vi "ReCheckStrips.vi"(0 "Probe Card Channels":i32=32, 5 "Auto Re-Check":bool, 7 "Thresholds":T1, 9 "Bad channel list":i32[](array[numeric]), 10 "region in":u32, 11 "Number of strips probed":i32) -> (3 "Thresholds copy":T2 {"Hi R" format="%.2f"; "Lo R" format="%.2f"; "Current threshold" format="%.1f"; "Lo Cap" format="%.2f"; "Hi Cap" format="%.2f"})   [LabVIEW 2018]
uses:
  InstrControl/SupplyControl/SupplyControl.lvclass
  ProbePlan/ProbePlanParams.vi
  InstrControl/Switching/Switching.lvclass
  InstrControl/LCRControl/LCRControl.lvclass
  general_VIs/globals/QC_MeasurementSetup.vi
  InstrControl/ProbeStationControl/ProbeStationControl.lvclass
panel:
  out "Current Bias Voltage [V]":dbl
  out "Bias On/Off:":bool
  out "Single Needle":bool
  out "Strip Offset":i32
  in  "min scale array":i32[](array[numeric])
  in  "max scale array":i32[](array[numeric])
  out "Current [nA]":cluster{u32, i32, "Array OUT":dbl[]}(graph)
  out "Capacitance [pF]":cluster{u32, i32, "Array OUT":dbl[]}(graph)
  out "Resistance [MW]":cluster{u32, i32, "Array OUT":dbl[]}(graph)
  out "Region:":string
  out "Defects":string
  out "old R Data":dbl format="%.2f"
  out "Resistance":dbl format="%.2f"
  in  "go/stop":bool
  in  "Mode:":u16(ring) items=["Remeasure defect list", "Remeasure cursor strip"]
  in  "Edit Mode:":u16(ring) items=["Manual", "Automatic"]
  out "old flag":u16(ring) items=["Not known", "OK", "Pinhole", "Punchthrough", "Short", "Open", "Resistor", "Implant"]
  out "new flag":u16(ring) items=["Not yet known", "OK", "Pinhole", "Punchthrough", "Short", "Open", "Resistor", "Implant"]
  in  "Cursor Plot:":u16(ring) items=["Current", "Capacitance", "Resistance"]
  out "old C data":dbl format="%.2f"
  out "old I data":dbl format="%.2f"
  out "No. of strips checked":i32
  out "this strip no.":i32
  in  "update list":bool
  in  "Quit":bool
  out "Capacitance":dbl format="%.2f"
  out "Current":dbl format="%.2f"
  in  "skip this strip":bool
  in  "Correct Data":bool
  in  "Read":bool
  out "No. of bad channels":i32
  # "Analysis / Remeasurement of Strip Data"
  # "Current [nA]"
  # "Capacitance [pF]"
  # "Resistance [MW]"
  # "Thresholds"
  # "Measurements"
  # "Read / Edit Data"
  # "New Data                Old Data"
  # "No. checked:"
  # "Current:"
  # "Capacitance:"
  # "This Strip:"
  # "Resistance:"
  # "Defect?"
  # "Defect Channels"
  # "Number:"
  # "Current [nA]:"
  # "Capacitance [pF]:"
  # "Resistance [MW]:"
  # "Low              High"
  # "Current:"
  # "nA"
  # "Capacitance:"
  # "pF"
  # "Resistance:"
  # "Mohm"
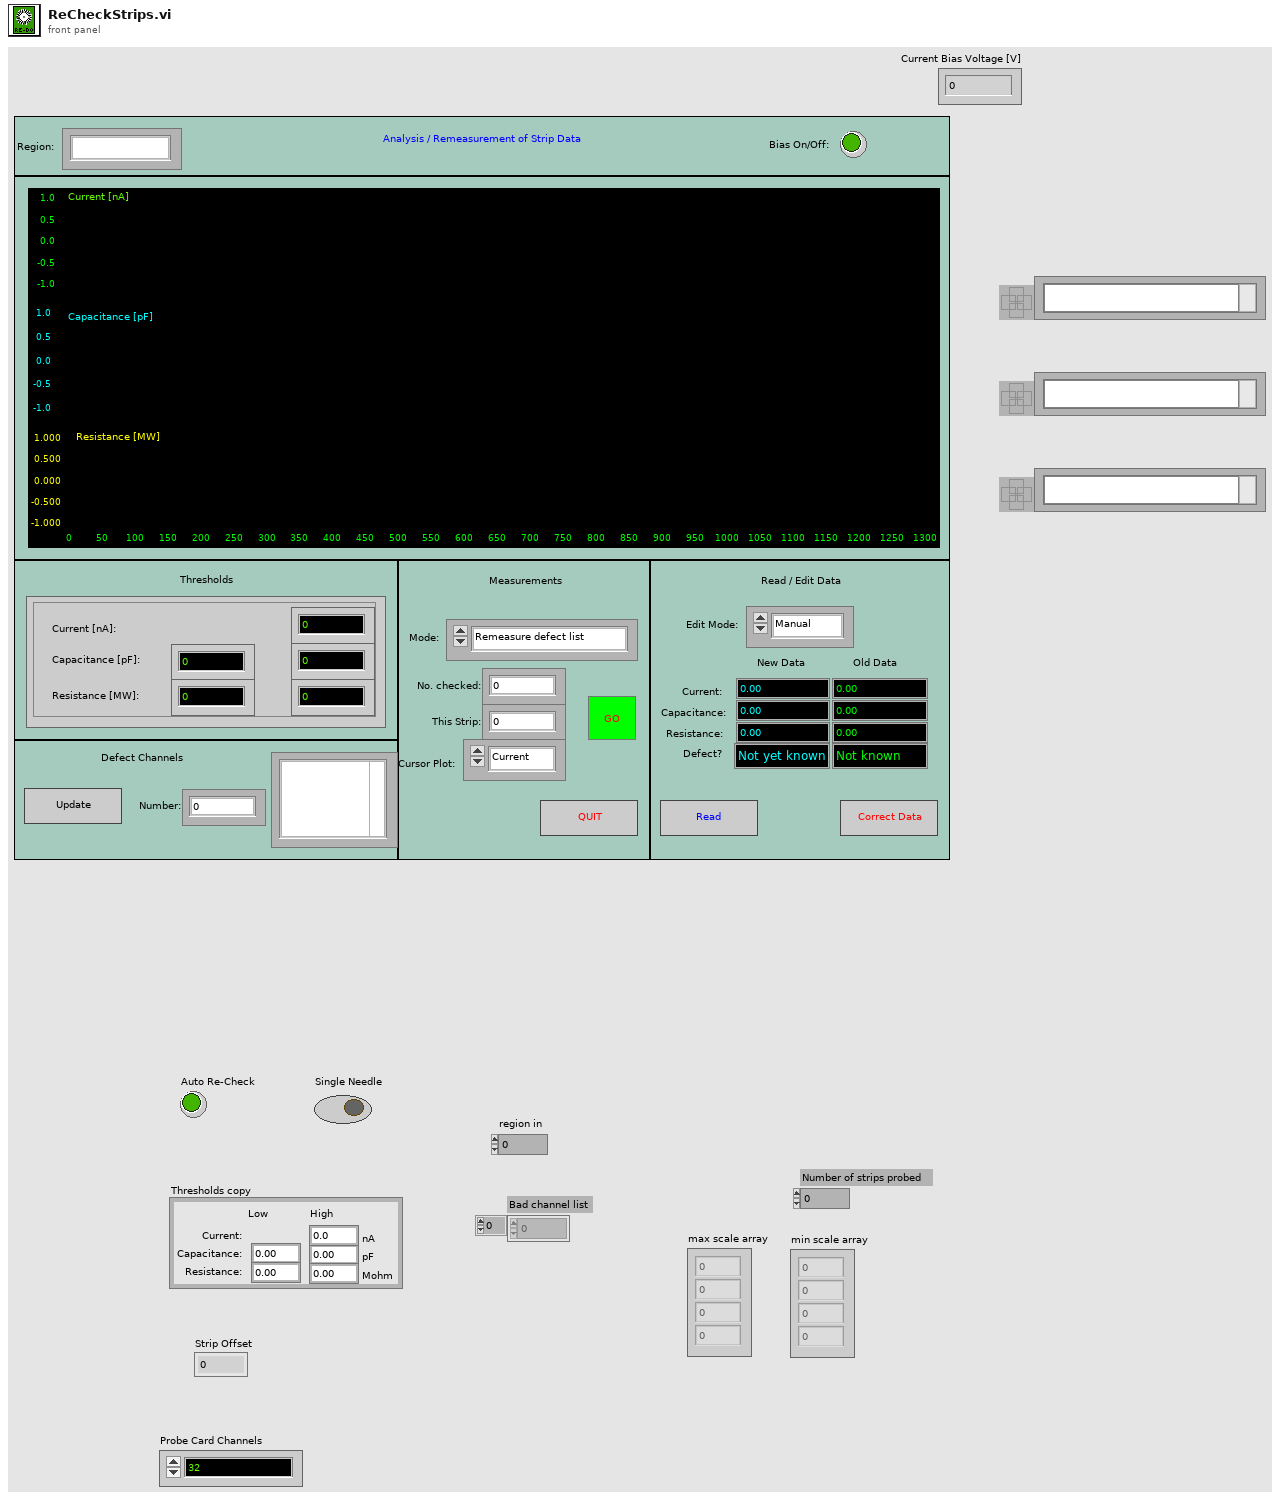
[diagram p1: front panel]
types:
  T1 = cluster{"Current [nA]":dbl, "Cap_Lo":dbl, "Cap_Hi":dbl, "Res_Hi":dbl, "Res_Lo":dbl}
  T2 = cluster{"Hi Cap":dbl, "Lo Cap":dbl, "Current threshold":dbl, "Lo R":dbl, "Hi R":dbl}
  T3 = cluster{"Strip Number OUT":i32, "X0":i32, "Y0":i32, "X1":i32, "Y1":i32, "Xref":dbl, "Yref":dbl, "ProbePlan type":u32, "Inner pads offset":ext, "Outer pads offset":ext, "l_inner":ext, "l_outer":ext, "strip numbering":u16, "Device Orientation":ext, "Stagger offset":i32, "Yoffset":dbl, "Strip pitch":dbl, "Fiducail separation":dbl, "Radius":ext, "Relative strip angles":dbl, "Probeplan description":string, "ProbePlan array":cluster{"Region":string, "ProbePoints":cluster{"X":dbl, "Y":dbl, "Label":string, "CardViable?":bool}[]}[], "Test ProbePoints":cluster{"Regions Enabled":bool[], "From index":u32[], "To index":u32[], "Strip length [cm]":dbl[]}}
  T4 = cluster{"Region":string, "ProbePoints":cluster{"X":dbl, "Y":dbl, "Label":string, "CardViable?":bool}[]}[]
  T5 = cluster{"Region":string, "ProbePoints":cluster{"X":dbl, "Y":dbl, "Label":string, "CardViable?":bool}[]}
  T6 = enum16{"Reset", "Ground", "Striptest SMU", "Striptest LCR", "IV", "CV", "Interstrip Cap", "Interstrip Res"}
  T7 = cluster{"Bias Supply":refnum<class "SupplyControl.lvclass">, "SMU":refnum<class "SupplyControl.lvclass">, "LCR":refnum<class "LCRControl.lvclass">, "ProbeStation":refnum<class "ProbeStationControl.lvclass">, "Arduino":refnum<class "ArduinoControl.lvclass">, "Measurement switch":refnum<class "Switching.lvclass">, "Probe Card Channels":i32, "Bias Voltage [V]":dbl, "First strip":i32, "Last strip":i32, "Base Voltage [V]":dbl, "Base Ramp Step [V]":dbl, "Base Ramp Interval [ms]":u32, "High Voltage [V]":dbl, "High Ramp Step [V]":dbl, "High Ramp Interval [ms]":u32, "AC frequency [Hz]":i32, "AC amplitude [V]":dbl, "RC Configuration":u16, "Single Needle":bool, "Temperature Readout":enum16{"Read Arduino", "Enter manually"}, "Fraction of good strips [%]":dbl, "Measurement switch used?":bool, "Matrix X Channels":cluster{"Mux1 C1":i32, "Mux1 C2":i32, "Mux2 C1":i32, "Mux2 C2":i32}, "Pinholes Y/N":bool, "Capacitance Y/N":bool, "Resistance Y/N":bool, "Bias Supply Name":string, "SMU Name":string, "LCR Name":string}
  T8 = cluster{"pass Rate in %":dbl, "Bad channel list":i32[], "No of bad strips":i32, "Defect description list":i32[], "Number of defects per category":i32[], "Defect lists":string[], "No of channels":i32, "Defect Flag array OUT":i32[][]}
  T9 = enum16{"Reset", "Read Array", "Read Element", "Write Element", "Write Array", "Add Element", "Add Array"}
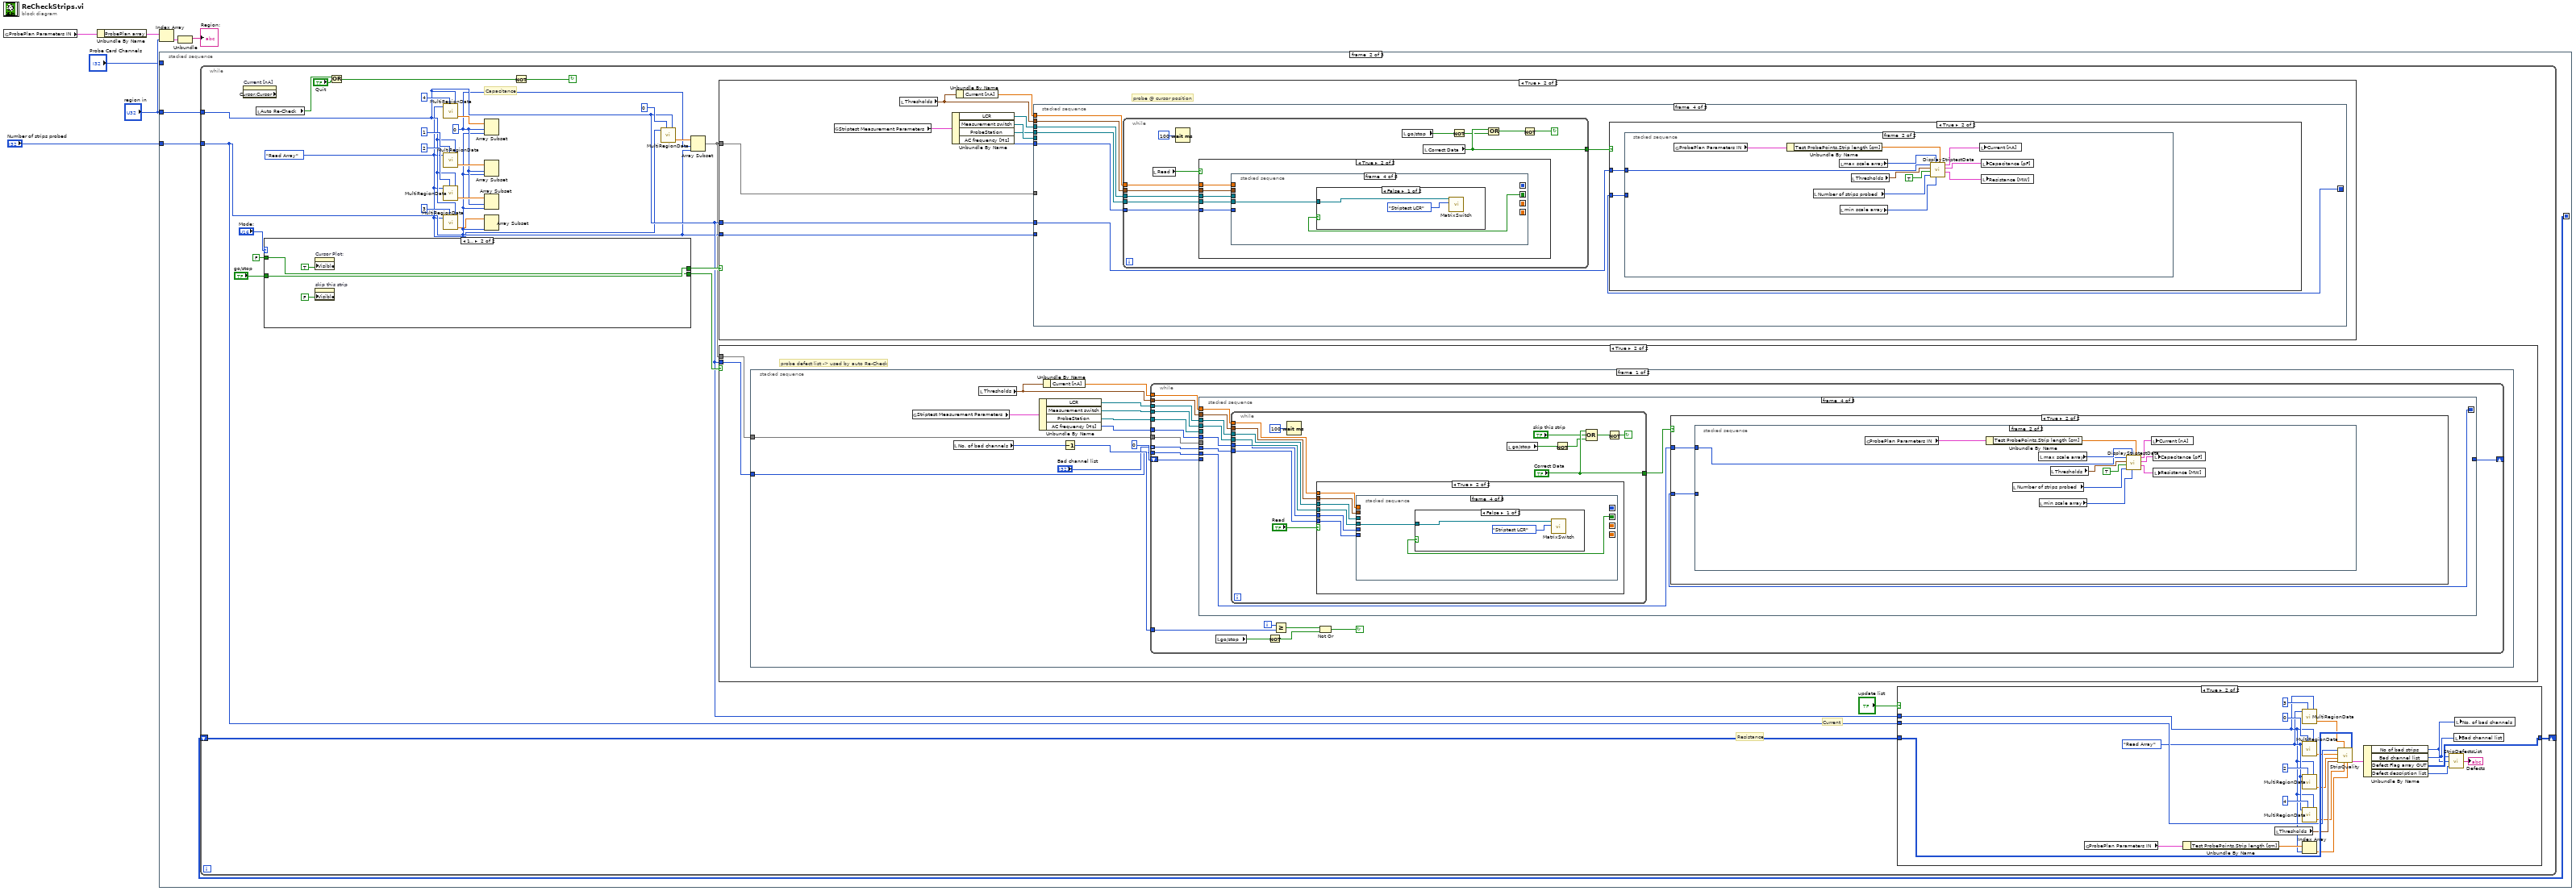
[diagram p0: block diagram]
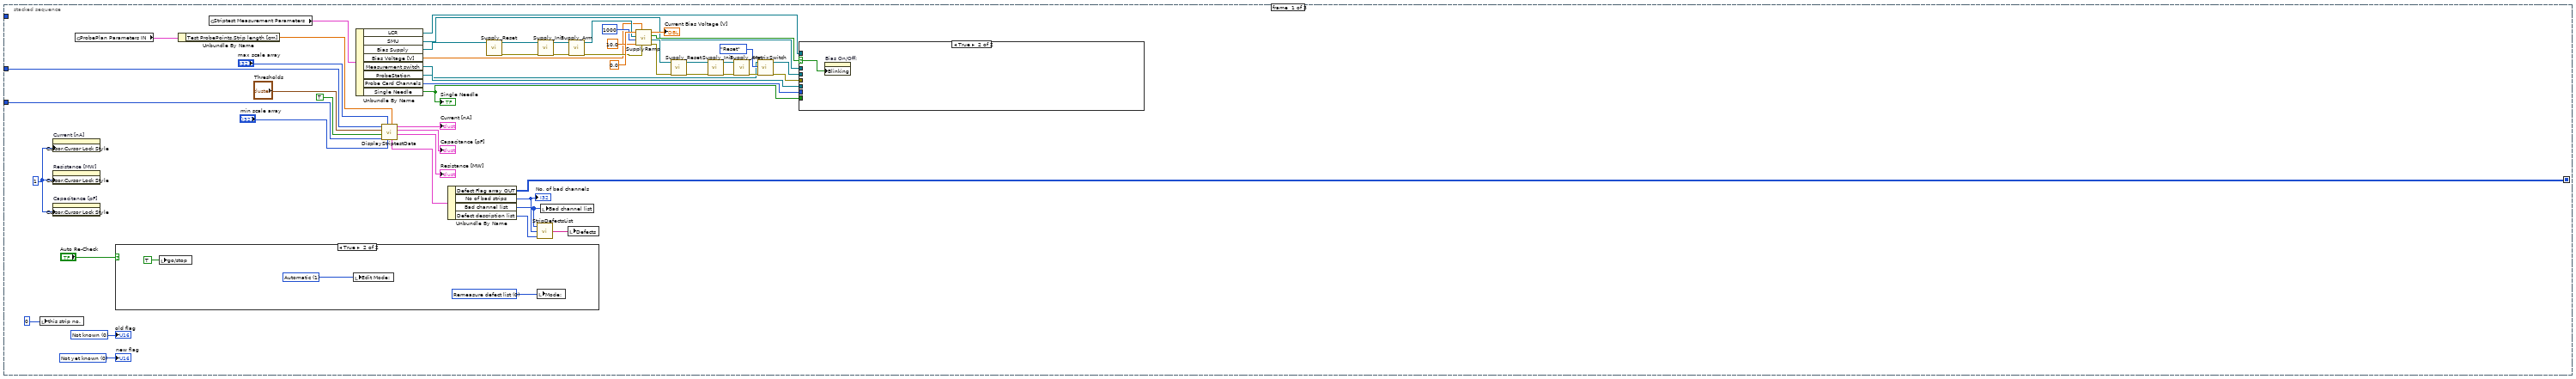
[diagram p2: hidden frame]
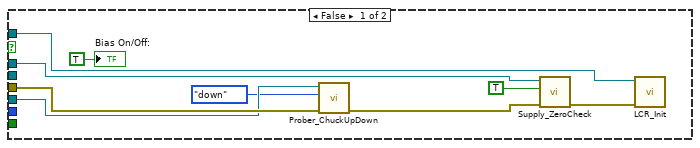
[diagram p3: hidden frame]
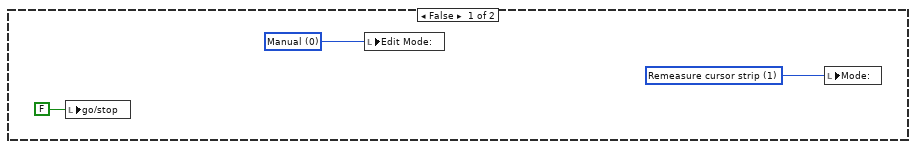
[diagram p4: hidden frame]
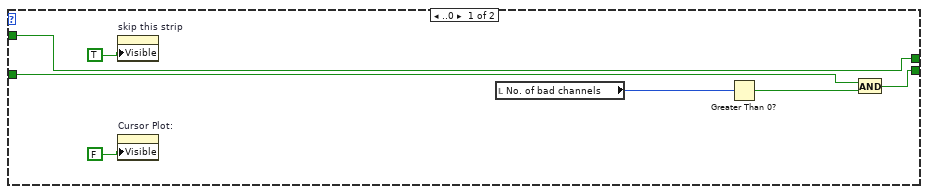
[diagram p5: hidden frame]
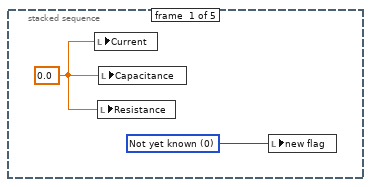
[diagram p7: hidden frame]
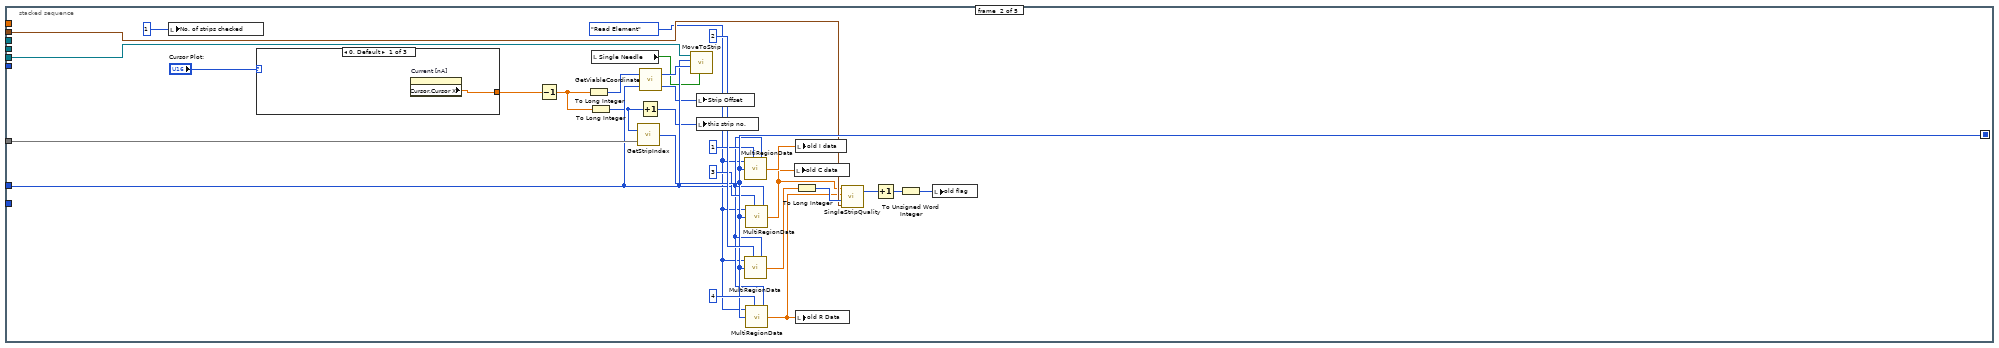
[diagram p8: hidden frame]
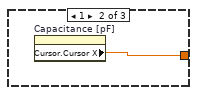
[diagram p9: hidden frame]
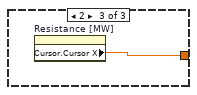
[diagram p10: hidden frame]
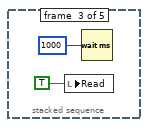
[diagram p11: hidden frame]
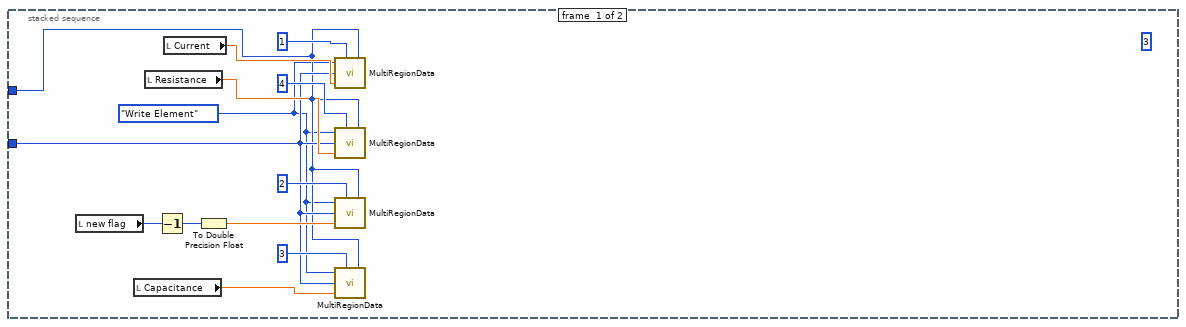
[diagram p13: hidden frame]
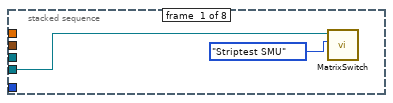
[diagram p15: hidden frame]
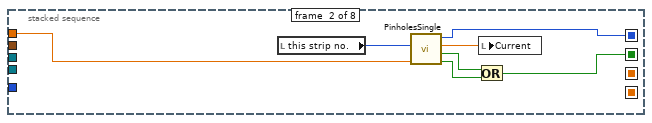
[diagram p16: hidden frame]
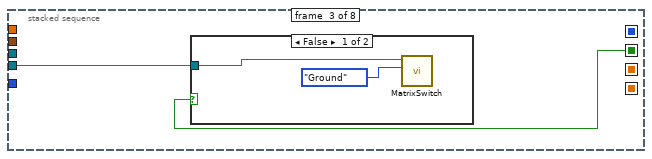
[diagram p17: hidden frame]
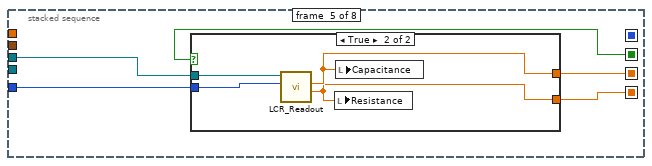
[diagram p20: hidden frame]
diagram:
  n1 = global read "ProbePlanParams.vi" "ProbePlan Parameters IN"() -> (w6:T3)
  n2 = Unbundle By Name(w6) -> ("ProbePlan array"=w5:T4)
  n3 = Index Array(array=w5, index="region in") -> (element=w3:T5)
  n4 = stacked-sequence {
    seq-local: [w58 _ _] -> [_ w76 _]
    tunnel: "Number of strips probed" -> [w48 w78 _]
    tunnel: "region in" -> [w50 w77 _]
    tunnel: "Probe Card Channels" -> [_ _ _]
    frame #0 {
      w55 = u16 0 items=["Not known", "OK", "Pinhole", "Punchthrough", "Short", "Open", "Resistor", "Implant"] ("old flag")
      w56 = u16 0 items=["Not yet known", "OK", "Pinhole", "Punchthrough", "Short", "Open", "Resistor", "Implant"] ("new flag")
      w44 = u32 1 ("Cursor Locked")
      n5 = local write "this strip no."(0 ("Current copy")) -> ()
      n6 = property on="Current [nA]" class="WFGraph (strict)"("Cursor.Cursor Lock Style"=w44) -> ()  [unwired: 2 in, 2 out]
      n7 = property on="Resistance [MW]" class="WFGraph (strict)"("Cursor.Cursor Lock Style"=w44) -> ()  [unwired: 2 in, 2 out]
      n8 = property on="Capacitance [pF]" class="WFGraph (strict)"("Cursor.Cursor Lock Style"=w44) -> ()  [unwired: 2 in, 2 out]
      n9 = global read "ProbePlanParams.vi" "ProbePlan Parameters IN"() -> (w9:T3)
      n10 = case shown="True" "Auto Re-Check" {
        frame False {
          w70 = u16 0 items=["Manual", "Automatic"] ("Edit Mode:")
          w71 = u16 1 items=["Remeasure defect list", "Remeasure cursor strip"] ("Mode:")
          n11 = local write "go/stop"(FALSE ("Check strips")) -> ()
          n12 = local write "Edit Mode:"(w70) -> ()
          n13 = local write "Mode:"(w71) -> ()
        }
        frame True {
          w74 = u16 1 items=["Manual", "Automatic"] ("Edit Mode:")
          w75 = u16 0 items=["Remeasure defect list", "Remeasure cursor strip"] ("Mode:")
          n14 = local write "go/stop"(TRUE ("Check strips")) -> ()
          n15 = local write "Edit Mode:"(w74) -> ()
          n16 = local write "Mode:"(w75) -> ()
        }
      }
      n17 = Unbundle By Name(w9) -> ("Test ProbePoints.Strip length [cm]"=w8:dbl[])
      n18 = global read "QC_MeasurementSetup.vi" "Striptest Measurement Parameters"() -> (w10:T7)
      n19 = Unbundle By Name(w10) -> ("LCR"=w16:refnum<class "LCRControl.lvclass">, "SMU"=w17:refnum<class "SupplyControl.lvclass">, "Bias Supply"=w18:refnum<class "SupplyControl.lvclass">, "Bias Voltage [V]"=w28:dbl, "Measurement switch"=w13:refnum<class "Switching.lvclass">, "ProbeStation"=w15:refnum<class "ProbeStationControl.lvclass">, "Probe Card Channels"=w12:i32, "Single Needle"=w11:bool)
      "Single Needle" <- w11
      n20 = call "DisplayStriptestData.vi"("Strip Lengths [cm]"=w8, "min scale array"="min scale array", "max scale array"="max scale array", "# probed"=w48, "Display Stats?"=TRUE, "Thresholds:"="Thresholds", "Region"=w50) -> ("Resistance [MW]"=→"Resistance [MW]":cluster{u32, i32, "Array OUT":dbl[]}, "Capacitance [pF]"=→"Capacitance [pF]":cluster{u32, i32, "Array OUT":dbl[]}, "Current [nA]"=→"Current [nA]":cluster{u32, i32, "Array OUT":dbl[]}, "Strip Quality Data"=w54:T8)  [unwired: 1 out]
      n21 = Unbundle By Name(w54) -> ("Defect Flag array OUT"=w58:i32[][], "No of bad strips"=w52:i32, "Bad channel list"=w51:i32[], "Defect description list"=w53:i32[])
      "No. of bad channels" <- w52
      n22 = call-dynamic "Supply_Reset.vi"("SupplyControl in"=w18) -> ("error out"=w32:errorcluster, "SupplyControl out"=w35:refnum<class "SupplyControl.lvclass">)  [unwired: 9 in]
      n23 = call "StripDefectsList.vi"("Defect description list"=w53, "No of strips"=w52, "Bad channel list"=w51) -> ("Defect list"=w57:string)
      n24 = call-dynamic "Supply_Init.vi"("error in (no error)"=w32, "SupplyControl in"=w35) -> ("error out"=w33:errorcluster, "SupplyControl out"=w34:refnum<class "SupplyControl.lvclass">)  [unwired: 8 in]
      n25 = local write "Bad channel list"(w51) -> ()
      n26 = local write "Defects"(w57) -> ()
      n27 = call-dynamic "Supply_Arm.vi"("error in (no error)"=w33, "SupplyControl in"=w34) -> ("error out"=w30:errorcluster, "SupplyControl out"=w31:refnum<class "SupplyControl.lvclass">)  [unwired: 8 in]
      n28 = call "SupplyRamp.vi"("error in"=w30, "Requested Voltage"=w28, "Step Size"=10.0, "Step Delay"=1000, "Supply IN"=w31, "Starting Voltage"=0.0) -> ("error out"=w29:errorcluster, "Supply OUT"=w14:refnum<class "SupplyControl.lvclass">, "Compliance exceeded"=w22:bool, "Current Voltage"=→"Current Bias Voltage [V]":dbl)  [unwired: 2 in]
      n29 = call-dynamic "Supply_Reset.vi"("error in (no error)"=w29, "SupplyControl in"=w17) -> ("error out"=w26:errorcluster, "SupplyControl out"=w25:refnum<class "SupplyControl.lvclass">)  [unwired: 8 in]
      n30 = call-dynamic "Supply_Init.vi"("error in (no error)"=w26, "SupplyControl in"=w25) -> ("error out"=w27:errorcluster, "SupplyControl out"=w24:refnum<class "SupplyControl.lvclass">)  [unwired: 8 in]
      n31 = call-dynamic "Supply_Arm.vi"("error in (no error)"=w27, "SupplyControl in"=w24) -> ("error out"=w39:errorcluster)  [unwired: 8 in, 1 out]
      n32 = call-dynamic "MatrixSwitch.vi"("error in (no error)"=w39, "Action"=T6."Reset", "Switching in"=w13) -> ("error out"=w19:errorcluster, "Switching out"=w20:refnum<class "Switching.lvclass">)  [unwired: 6 in, 1 out]
      n33 = case shown="True" w22 {
        selector: w22 -> [_ w69]
        tunnel: w20 -> [_ _]
        tunnel: w19 -> [w68 _]
        tunnel: w16 -> [w65 _]
        tunnel: w15 -> [w67 _]
        tunnel: w14 -> [w64 _]
        tunnel: w12 -> [_ _]
        tunnel: w11 -> [_ _]
        frame False {
          n34 = call-dynamic "Prober_ChuckUpDown.vi"("error in (no error)"=w68, "Direction"=enum16{"up", "down"}."down", "ProbeStationControl in"=w67) -> ("error out"=w63:errorcluster)  [unwired: 6 in, 2 out]
          n35 = call-dynamic "Supply_ZeroCheck.vi"("error in (no error)"=w63, "enable/disable"=TRUE, "SupplyControl in"=w64) -> ("error out"=w60:errorcluster)  [unwired: 7 in, 1 out]
          n36 = call-dynamic "LCR_Init.vi"("error in (no error)"=w60, "LCRControl in"=w65) -> ()  [unwired: 8 in, 2 out]
          "Bias On/Off:" <- TRUE ("Bias On?")
        }
        frame True {
          n37 = property on="Bias On/Off:" class="Bool (strict)"("Blinking"=w69) -> ()  [unwired: 2 in, 2 out]
        }
      }
      "new flag" <- w56
      "old flag" <- w55
    }
    frame #1 {
      n38 = while {
        shift-right: [w100] -> _
        shift-left: w76 -> [w98]
        tunnel: w78 -> [w85]
        tunnel: w77 -> [w92]
        stop <- w105 continue-if-true
        w79 = T9."Read Array" ("Action")
        w86 = 0
        # "Resistance"
        # "Capacitance"
        # "Current"
        n39 = property on="Current [nA]" class="WFGraph (strict)" props=["Cursor", "Cursor X"]() -> ()  [unwired: 2 in, 3 out]
        n40 = local read "Auto Re-Check"() -> (w82:bool)
        n41 = case shown="1.." "Mode:" {
          tunnel: "go/stop" -> [w110 w116]
          tunnel: [w109 w115] -> w103
          tunnel: [w108 w116] -> w102
          tunnel: FALSE -> [w108 w115]
          frame ..0 {
            n42 = property on="skip this strip" class="Bool"("Visible"=TRUE) -> ()  [unwired: 2 in, 2 out]
            n43 = property on="Cursor Plot:" class="Ring (strict)"("Visible"=FALSE) -> ()  [unwired: 2 in, 2 out]
            n44 = local read "No. of bad channels"() -> (w112:i32)
            n45 = Greater Than 0?(x=w112) -> (x > 0?=w111:bool)
            n46 = And(x=w110, y=w111) -> (x .and. y?=w109:bool)
          }
          frame 1.. {
            n47 = property on="Cursor Plot:" class="Ring (strict)"("Visible"=TRUE) -> ()  [unwired: 2 in, 2 out]
            n48 = property on="skip this strip" class="Bool"("Visible"=FALSE) -> ()  [unwired: 2 in, 2 out]
          }
        }
        n49 = Or(x=w82, y="Quit") -> (x .or. y?=w80:bool)
        n50 = call "MultiRegionData.vi"("Action"=w79, "Array No."=4, "Region index"=w92) -> ("Array OUT"=w90:dbl[])  [unwired: 3 in, 1 out]
        n51 = call "MultiRegionData.vi"("Action"=w79, "Array No."=1, "Region index"=w92) -> ("Array OUT"=w89:dbl[])  [unwired: 3 in, 1 out]
        n52 = call "MultiRegionData.vi"("Action"=w79, "Array No."=2, "Region index"=w92) -> ("Array OUT"=w88:dbl[])  [unwired: 3 in, 1 out]
        n53 = call "MultiRegionData.vi"("Action"=w79, "Array No."=3, "Region index"=w92) -> ("Array OUT"=w87:dbl[])  [unwired: 3 in, 1 out]
        n54 = Array Subset(array=w90, index=w86, length=w85) -> ()  [unwired: 1 out]
        n55 = Array Subset(array=w89, index=w86, length=w85) -> ()  [unwired: 1 out]
        n56 = Array Subset(array=w88, index=w86, length=w85) -> ()  [unwired: 1 out]
        n57 = Array Subset(array=w87, length=w85) -> ()  [unwired: 1 in, 1 out]
        n58 = Not(x=w80) -> (.not. x?=w105:bool)
        n59 = call "MultiRegionData.vi"("Action"=w79, "Array No."=0, "Region index"=w92) -> ("Array OUT"=w91:dbl[])  [unwired: 3 in, 1 out]
        n60 = Array Subset(array=w91, index=w86, length=w85) -> (w84:dbl[])
        n61 = case shown="True" w102 {
          tunnel: w84 -> [_ w126]
          tunnel: w85 -> [_ w123]
          tunnel: w92 -> [_ w122]
          frame False {
          }
          frame True {
            # "probe @ cursor position"
            n62 = global read "QC_MeasurementSetup.vi" "Striptest Measurement Parameters"() -> (w121:T7)
            n63 = local read "Thresholds"() -> (w124:T1)
            n64 = Unbundle By Name(w121) -> ("LCR"=w117:refnum<class "LCRControl.lvclass">, "Measurement switch"=w119:refnum<class "Switching.lvclass">, "ProbeStation"=w120:refnum<class "ProbeStationControl.lvclass">, "AC frequency [Hz]"=w118:i32)
            n65 = Unbundle By Name(w124) -> ("Current [nA]"=w125:dbl)
            n66 = stacked-sequence {
              seq-local: [_ w150 _ _ _] -> [_ _ _ w168 _]
              tunnel: w126 -> [_ w153 _ _ _]
              tunnel: w125 -> [_ _ _ w167 _]
              tunnel: w124 -> [_ w145 _ w166 _]
              tunnel: w123 -> [_ _ _ _ _]
              tunnel: w122 -> [_ w137 _ w165 _]
              tunnel: w120 -> [_ w131 _ _ _]
              tunnel: w119 -> [_ _ _ w164 _]
              tunnel: w118 -> [_ _ _ w163 _]
              tunnel: w117 -> [_ _ _ w162 _]
              frame #0 {
                w127 = u16 0 items=["Not yet known", "OK", "Pinhole", "Punchthrough", "Short", "Open", "Resistor", "Implant"] ("new flag")
                w128 = 0.0 ("Current")
                n67 = local write "Current"(w128) -> ()
                n68 = local write "Resistance"(w128) -> ()
                n69 = local write "Capacitance"(w128) -> ()
                n70 = local write "new flag"(w127) -> ()
              }
              frame #1 {
                w129 = T9."Read Element" ("Action")
                n71 = local write "No. of strips checked"(1 ("Current copy 2")) -> ()
                n72 = case shown="0, Default" "Cursor Plot:" {
                  tunnel: [w157 w158 w159] -> w135
                  frame 0, Default {
                    n73 = property on="Current [nA]" class="WFGraph (strict)"() -> ("Cursor.Cursor X"=w157:dbl)  [unwired: 2 in, 2 out]
                  }
                  frame 1 {
                    n74 = property on="Capacitance [pF]" class="WFGraph (strict)"() -> ("Cursor.Cursor X"=w158:dbl)  [unwired: 2 in, 2 out]
                  }
                  frame 2 {
                    n75 = property on="Resistance [MW]" class="WFGraph (strict)"() -> ("Cursor.Cursor X"=w159:dbl)  [unwired: 2 in, 2 out]
                  }
                }
                n76 = Decrement(x=w135) -> (x-1=w134:dbl)
                n77 = To Long Integer(number=w134) -> (32bit integer=w138:i32)
                n78 = To Long Integer(number=w134) -> (32bit integer=w133:i32)
                n79 = local read "Single Needle"() -> (w130:bool)
                n80 = call "GetStripIndex.vi"("Channel no array in"=w153, "Channel no. in"=w133) -> ("Index out"=w150:i32)
                n81 = call "GetViableCoordinate.vi"("Target Region [0-3]"=w137, "Actual Target Strip [0-1279]"=w138) -> ("Offset"=w136:i32, "Move Probecard to Strip #"=w139:i32)
                n82 = Increment(x=w133) -> (x+1=w132:i32)
                n83 = call "MoveToStrip.vi"("Single Needle"=w130, "Strip No."=w139, "Region"=w137, "ProbeStationControl in"=w131) -> ()  [unwired: 5 in, 3 out]
                n84 = local write "Strip Offset"(w136) -> ()
                n85 = local write "this strip no."(w132) -> ()
                n86 = call "MultiRegionData.vi"("Action"=w129, "Array No."=1, "Array Size / Index"=w150, "Region index"=w137) -> ("Data OUT"=w156:dbl)  [unwired: 2 in, 1 out]
                n87 = call "MultiRegionData.vi"("Action"=w129, "Array No."=2, "Array Size / Index"=w150, "Region index"=w137) -> ("Data OUT"=w149:dbl)  [unwired: 2 in, 1 out]
                n88 = call "MultiRegionData.vi"("Action"=w129, "Array No."=3, "Array Size / Index"=w150, "Region index"=w137) -> ("Data OUT"=w144:dbl)  [unwired: 2 in, 1 out]
                n89 = call "MultiRegionData.vi"("Action"=w129, "Array No."=4, "Array Size / Index"=w150, "Region index"=w137) -> ("Data OUT"=w143:dbl)  [unwired: 2 in, 1 out]
                n90 = local write "old C data"(w144) -> ()
                n91 = local write "old I data"(w156) -> ()
                n92 = local write "old R Data"(w143) -> ()
                n93 = To Long Integer(number=w149) -> (32bit integer=w148:i32)
                n94 = call "SingleStripQuality.vi"("Thresholds"=w145, "Pinhole flag in"=w148, "Resistance Data"=w143, "Capacitance Data"=w144) -> ("Defect Flag"=w142:i32)  [unwired: 2 in, 1 out]
                n95 = Increment(x=w142) -> (x+1=w141:i32)
                n96 = To Unsigned Word Integer(number=w141) -> (unsigned 16bit integer=w140:u16)
                n97 = local write "old flag"(w140) -> ()
              }
              frame #2 {
                n98 = local write "Read"(TRUE) -> ()
                n99 = Wait (ms)(milliseconds to wait=u32 1000 ("millisecond timer value")) -> ()  [unwired: 1 out]
              }
              frame #3 {
                n100 = while {
                  tunnel: [w203] -> w169
                  tunnel: w167 -> [w200]
                  tunnel: w166 -> [w199]
                  tunnel: w163 -> [w198]
                  tunnel: w164 -> [w197]
                  tunnel: w162 -> [w196]
                  stop <- w205 continue-if-true
                  n101 = local read "Read"() -> (w204:bool)
                  n102 = Wait (ms)(milliseconds to wait=100) -> ()  [unwired: 1 out]
                  n103 = case shown="True" w204 {
                    tunnel: w200 -> [_ w212]
                    tunnel: w199 -> [_ w211]
                    tunnel: w198 -> [_ w210]
                    tunnel: w197 -> [_ w209]
                    tunnel: w196 -> [_ w208]
                    frame False {
                    }
                    frame True {
                      n104 = stacked-sequence {
                        seq-local: [_ w220 _ _ _ _ _ _] -> [_ _ _ _ _ w247 _ _]
                        seq-local: [_ _ _ _ w234 _ _ _] -> [_ _ _ _ _ w246 _ _]
                        seq-local: [_ _ _ _ w233 _ _ _] -> [_ _ _ _ _ w245 _ _]
                        seq-local: [_ w216 _ _ _ _ _ _] -> [_ _ w223 w227 w231 _ _ _]
                        tunnel: w212 -> [_ w221 _ _ _ _ _ _]
                        tunnel: w211 -> [_ _ _ _ _ w244 _ _]
                        tunnel: w210 -> [_ _ _ _ w232 _ _ _]
                        tunnel: w209 -> [w213 _ w222 w226 _ _ _ _]
                        tunnel: w208 -> [_ _ _ _ w230 _ _ _]
                        frame #0 {
                          n105 = call-dynamic "MatrixSwitch.vi"("Action"=T6."Striptest SMU", "Switching in"=w213) -> ()  [unwired: 7 in, 3 out]
                        }
                        frame #1 {
                          n106 = local read "this strip no."() -> (w215:i32)
                          n107 = call "PinholesSingle.vi"("Current Threshold [nA]"=w221, "Channel"=w215) -> ("Compliance?"=w218:bool, "channel excluded"=w217:bool, "Current [nA]"=w219:dbl, "Flag"=w220:i32)  [unwired: 2 in]
                          n108 = Or(x=w217, y=w218) -> (x .or. y?=w216:bool)
                          n109 = local write "Current"(w219) -> ()
                        }
                        frame #2 {
                          n110 = case shown="False" w223 {
                            tunnel: w222 -> [w225 _]
                            frame False {
                              n111 = call-dynamic "MatrixSwitch.vi"("Action"=T6."Ground", "Switching in"=w225) -> ()  [unwired: 7 in, 3 out]
                            }
                            frame True {
                            }
                          }
                        }
                        frame #3 {
                          n112 = case shown="False" w227 {
                            tunnel: w226 -> [w229 _]
                            frame False {
                              n113 = call-dynamic "MatrixSwitch.vi"("Action"=T6."Striptest LCR", "Switching in"=w229) -> ()  [unwired: 7 in, 3 out]
                            }
                            frame True {
                            }
                          }
                        }
                        frame #4 {
                          n114 = case shown="True" w231 {
                            tunnel: [w235 w240] -> w234
                            tunnel: [w236 w239] -> w233
                            tunnel: w232 -> [_ w238]
                            tunnel: w230 -> [_ w237]
                            frame False {
                              n115 = local read "old R Data"() -> (w236:dbl)
                              n116 = local read "old C data"() -> (w235:dbl)
                            }
                            frame True {
                              n117 = call-dynamic "LCR_Readout.vi"(10:w238, "LCRControl in"=w237) -> ("Resistance in Ohm"=w239:dbl, "Capacitance in pF"=w240:dbl)  [unwired: 6 in, 2 out]
                              n118 = local write "Resistance"(w239) -> ()
                              n119 = local write "Capacitance"(w240) -> ()
                            }
                          }
                        }
                        frame #5 {
                          n120 = call "SingleStripQuality.vi"("Thresholds"=w244, "Pinhole flag in"=w247, "Resistance Data"=w245, "Capacitance Data"=w246) -> ("Defect Flag"=w243:i32)  [unwired: 2 in, 1 out]
                          n121 = Increment(x=w243) -> (x+1=w242:i32)
                          n122 = To Unsigned Word Integer(number=w242) -> (unsigned 16bit integer=w241:u16)
                          n123 = local write "new flag"(w241) -> ()
                        }
                        frame #6 {
                          n124 = local read "Edit Mode:"() -> (w249:u16)
                          n125 = Greater Than 0?(x=w249) -> (x > 0?=w248:bool)
                          n126 = local write "Correct Data"(w248) -> ()
                        }
                        frame #7 {
                          n127 = local write "Read"(FALSE ("Read")) -> ()
                        }
                      }
                    }
                  }
                  n128 = local read "go/stop"() -> (w202:bool)
                  n129 = local read "Correct Data"() -> (w203:bool)
                  n130 = Not(x=w202) -> (.not. x?=w201:bool)
                  n131 = Compound Arithmetic op=OR(w203, w201) -> (w206:bool)
                  n132 = Not(x=w206) -> (.not. x?=w205:bool)
                }
                n133 = case shown="True" w169 {
                  tunnel: w168 -> [_ w171]
                  tunnel: w165 -> [_ w170]
                  frame False {
                  }
                  frame True {
                    n134 = stacked-sequence {
                      tunnel: w171 -> [w174 _]
                      tunnel: w170 -> [w173 w192]
                      frame #0 {
                        w172 = T9."Write Element" ("Action")
                        (unwired) u32 3 ("Action")
                        n135 = local read "new flag"() -> (w178:u16)
                        n136 = local read "Capacitance"() -> (w182:dbl)
                        n137 = local read "Resistance"() -> (w179:dbl)
                        n138 = Decrement(x=w178) -> (x-1=w176:u16)
                        n139 = local read "Current"() -> (w181:dbl)
                        n140 = To Double Precision Float(number=w176) -> (double precision float=w177:dbl)
                        n141 = call "MultiRegionData.vi"("Action"=w172, "Array No."=1, "Array Size / Index"=w174, "Data IN"=w181, "Region index"=w173) -> ()  [unwired: 1 in, 2 out]
                        n142 = call "MultiRegionData.vi"("Action"=w172, "Array No."=4, "Array Size / Index"=w174, "Data IN"=w179, "Region index"=w173) -> ()  [unwired: 1 in, 2 out]
                        n143 = call "MultiRegionData.vi"("Action"=w172, "Array No."=2, "Array Size / Index"=w174, "Data IN"=w177, "Region index"=w173) -> ()  [unwired: 1 in, 2 out]
                        n144 = call "MultiRegionData.vi"("Action"=w172, "Array No."=3, "Array Size / Index"=w174, "Data IN"=w182, "Region index"=w173) -> ()  [unwired: 1 in, 2 out]
                      }
                      frame #1 {
                        n145 = global read "ProbePlanParams.vi" "ProbePlan Parameters IN"() -> (w186:T3)
                        n146 = Unbundle By Name(w186) -> ("Test ProbePoints.Strip length [cm]"=w185:dbl[])
                        n147 = local read "Number of strips probed"() -> (w191:i32)
                        n148 = local read "max scale array"() -> (w187:i32[])
                        n149 = local read "min scale array"() -> (w188:i32[])
                        n150 = local read "Thresholds"() -> (w189:T1)
                        n151 = call "DisplayStriptestData.vi"("Strip Lengths [cm]"=w185, "min scale array"=w188, "max scale array"=w187, "# probed"=w191, "Display Stats?"=TRUE, "Thresholds:"=w189, "Region"=w192) -> ("Resistance [MW]"=w193:cluster{u32, i32, "Array OUT":dbl[]}, "Capacitance [pF]"=w194:cluster{u32, i32, "Array OUT":dbl[]}, "Current [nA]"=w195:cluster{u32, i32, "Array OUT":dbl[]})  [unwired: 2 out]
                        n152 = local write "Current [nA]"(w195) -> ()
                        n153 = local write "Capacitance [pF]"(w194) -> ()
                        n154 = local write "Resistance [MW]"(w193) -> ()
                      }
                    }
                  }
                }
              }
              frame #4 {
                w251 = FALSE
                n155 = local write "Read"(w251) -> ()
                n156 = local write "go/stop"(w251) -> ()
                n157 = local write "Correct Data"(w251) -> ()
              }
            }
          }
        }
        n158 = case shown="True" w103 {
          tunnel: w84 -> [_ w253]
          tunnel: w92 -> [_ w252]
          frame False {
          }
          frame True {
            # "probe defect list -> used by auto Re-Check"
            n159 = stacked-sequence {
              tunnel: w253 -> [w263 _]
              tunnel: w252 -> [w259 _]
              frame #0 {
                n160 = global read "QC_MeasurementSetup.vi" "Striptest Measurement Parameters"() -> (w258:T7)
                n161 = local read "No. of bad channels"() -> (w265:i32)
                n162 = local read "Thresholds"() -> (w260:T1)
                n163 = Unbundle By Name(w258) -> ("LCR"=w255:refnum<class "LCRControl.lvclass">, "Measurement switch"=w257:refnum<class "Switching.lvclass">, "ProbeStation"=w254:refnum<class "ProbeStationControl.lvclass">, "AC frequency [Hz]"=w256:i32)
                n164 = Unbundle By Name(w260) -> ("Current [nA]"=w262:dbl)
                n165 = Decrement(x=w265) -> (x-1=w266:i32)
                n166 = while {
                  tunnel: "Bad channel list" -> [w272] mode=indexing
                  tunnel: w266 -> [w282]
                  shift-right: [w278] -> _
                  shift-left: 0 -> [w279]
                  tunnel: w262 -> [w277]
                  tunnel: w263 -> [w276]
                  tunnel: w260 -> [w273]
                  tunnel: w259 -> [w271]
                  tunnel: w257 -> [w270]
                  tunnel: w256 -> [w269]
                  tunnel: w255 -> [w268]
                  tunnel: w254 -> [w267]
                  i -> [w283]
                  stop <- w280 continue-if-true
                  n167 = stacked-sequence {
                    seq-local: [_ w291 _ _ _] -> [_ _ _ w330 _]
                    tunnel: w272 -> [_ w292 _ w326 _]
                    tunnel: w279 -> [_ w294 _ _ _]
                    tunnel: [_ w293 _ _ _] -> w278
                    tunnel: w277 -> [_ _ _ w329 _]
                    tunnel: w276 -> [_ w290 _ _ _]
                    tunnel: w273 -> [_ w288 _ w328 _]
                    tunnel: w271 -> [_ w287 _ w327 _]
                    tunnel: w270 -> [_ _ _ w325 _]
                    tunnel: w269 -> [_ _ _ w324 _]
                    tunnel: w268 -> [_ _ _ w323 _]
                    tunnel: w267 -> [_ w286 _ _ _]
                    frame #0 {
                      w284 = u16 0 items=["Not yet known", "OK", "Pinhole", "Punchthrough", "Short", "Open", "Resistor", "Implant"] ("new flag")
                      w285 = 0.0
                      n168 = local write "Current"(w285) -> ()
                      n169 = local write "Resistance"(w285) -> ()
                      n170 = local write "Capacitance"(w285) -> ()
                      n171 = local write "new flag"(w284) -> ()
                    }
                    frame #1 {
                      n172 = call "GetStripIndex.vi"("Channel no array in"=w290, "Channel no. in"=w292) -> ("Index out"=w291:i32)
                      n173 = local read "go/stop"() -> (w289:bool)
                      n174 = case shown="True" w289 {
                        tunnel: [w295 w319] -> w293
                        tunnel: w294 -> [w295 w318]
                        tunnel: w292 -> [_ w300]
                        tunnel: w291 -> [_ w304]
                        tunnel: w288 -> [_ w308]
                        tunnel: w287 -> [_ w303]
                        tunnel: w286 -> [_ w297]
                        frame False {
                        }
                        frame True {
                          w296 = T9."Read Element" ("Action")
                          n175 = Increment(x=w300) -> (x+1=→"this strip no.":i32)
                          n176 = call "GetViableCoordinate.vi"("Target Region [0-3]"=w303, "Actual Target Strip [0-1279]"=w300) -> ("Offset"=→"Strip Offset":i32, "Move Probecard to Strip #"=w302:i32)
                          n177 = Increment(x=w318) -> (x+1=w319:i32)
                          "No. of strips checked" <- w319
                          n178 = local read "Single Needle"() -> (w298:bool)
                          n179 = call "MoveToStrip.vi"("Single Needle"=w298, "Strip No."=w302, "Region"=w303, "ProbeStationControl in"=w297) -> ()  [unwired: 5 in, 3 out]
                          n180 = call "MultiRegionData.vi"("Action"=w296, "Array No."=2, "Array Size / Index"=w304, "Region index"=w303) -> ("Data OUT"=w310:dbl)  [unwired: 2 in, 1 out]
                          n181 = call "MultiRegionData.vi"("Action"=w296, "Array No."=1, "Array Size / Index"=w304, "Region index"=w303) -> ("Data OUT"=→"old I data":dbl)  [unwired: 2 in, 1 out]
                          n182 = call "MultiRegionData.vi"("Action"=w296, "Array No."=3, "Array Size / Index"=w304, "Region index"=w303) -> ("Data OUT"=w312:dbl)  [unwired: 2 in, 1 out]
                          "old C data" <- w312
                          n183 = call "MultiRegionData.vi"("Action"=w296, "Array No."=4, "Array Size / Index"=w304, "Region index"=w303) -> ("Data OUT"=w311:dbl)  [unwired: 2 in, 1 out]
                          "old R Data" <- w311
                          n184 = To Long Integer(number=w310) -> (32bit integer=w309:i32)
                          n185 = call "SingleStripQuality.vi"("Thresholds"=w308, "Pinhole flag in"=w309, "Resistance Data"=w311, "Capacitance Data"=w312) -> ("Defect Flag"=w307:i32)  [unwired: 2 in, 1 out]
                          n186 = Increment(x=w307) -> (x+1=w306:i32)
                          n187 = To Unsigned Word Integer(number=w306) -> (unsigned 16bit integer=w305:u16)
                          n188 = local write "old flag"(w305) -> ()
                        }
                      }
                    }
                    frame #2 {
                      n189 = local read "go/stop"() -> (w320:bool)
                      n190 = case shown="True" w320 {
                        frame False {
                        }
                        frame True {
                          n191 = local write "Read"(TRUE ("Read")) -> ()
                          n192 = Wait (ms)(milliseconds to wait=u32 1000) -> ()  [unwired: 1 out]
                        }
                      }
                    }
                    frame #3 {
                      n193 = while {
                        tunnel: ["Correct Data"] -> w331
                        tunnel: w329 -> [w365]
                        tunnel: w328 -> [w362]
                        tunnel: w326 -> [w361]
                        tunnel: w325 -> [w360]
                        tunnel: w324 -> [w359]
                        tunnel: w323 -> [w358]
                        stop <- w366 continue-if-true
                        n194 = Wait (ms)(milliseconds to wait=u32 100) -> ()  [unwired: 1 out]
                        n195 = case shown="True" "Read" {
                          tunnel: w365 -> [_ w377]
                          tunnel: w362 -> [_ w376]
                          tunnel: w361 -> [_ w375]
                          tunnel: w360 -> [_ w374]
                          tunnel: w359 -> [_ w373]
                          tunnel: w358 -> [_ w372]
                          frame False {
                          }
                          frame True {
                            n196 = stacked-sequence {
                              seq-local: [_ w385 _ _ _ _ _ _] -> [_ _ _ _ _ w412 _ _]
                              seq-local: [_ _ _ _ w399 _ _ _] -> [_ _ _ _ _ w411 _ _]
                              seq-local: [_ _ _ _ w398 _ _ _] -> [_ _ _ _ _ w410 _ _]
                              seq-local: [_ w381 _ _ _ _ _ _] -> [_ _ w388 w392 w396 _ _ _]
                              tunnel: w377 -> [_ w386 _ _ _ _ _ _]
                              tunnel: w376 -> [_ _ _ _ _ w409 _ _]
                              tunnel: w373 -> [_ _ _ _ w397 _ _ _]
                              tunnel: w375 -> [_ w380 _ _ _ _ _ _]
                              tunnel: w374 -> [w379 _ w387 w391 _ _ _ _]
                              tunnel: w372 -> [_ _ _ _ w395 _ _ _]
                              frame #0 {
                                n197 = call-dynamic "MatrixSwitch.vi"("Action"=T6."Striptest SMU", "Switching in"=w379) -> ()  [unwired: 7 in, 3 out]
                              }
                              frame #1 {
                                n198 = call "PinholesSingle.vi"("Current Threshold [nA]"=w386, "Channel"=w380) -> ("Compliance?"=w382:bool, "channel excluded"=w383:bool, "Current [nA]"=→"Current":dbl, "Flag"=w385:i32)  [unwired: 2 in]
                                n199 = Or(x=w383, y=w382) -> (x .or. y?=w381:bool)
                              }
                              frame #2 {
                                n200 = case shown="False" w388 {
                                tunnel: w387 -> [w390 _]
                                frame False {
                                n201 = call-dynamic "MatrixSwitch.vi"("Action"=T6."Ground", "Switching in"=w390) -> ()  [unwired: 7 in, 3 out]
                                }
                                frame True {
                                }
                                }
                              }
                              frame #3 {
                                n202 = case shown="False" w392 {
                                tunnel: w391 -> [w394 _]
                                frame False {
                                n203 = call-dynamic "MatrixSwitch.vi"("Action"=T6."Striptest LCR", "Switching in"=w394) -> ()  [unwired: 7 in, 3 out]
                                }
                                frame True {
                                }
                                }
                              }
                              frame #4 {
                                n204 = case shown="False" w396 {
                                tunnel: [w403 w404] -> w399
                                tunnel: [w402 w405] -> w398
                                tunnel: w397 -> [w401 _]
                                tunnel: w395 -> [w400 _]
                                frame False {
                                n205 = call-dynamic "LCR_Readout.vi"(10:w401, "LCRControl in"=w400) -> ("Resistance in Ohm"=w402:dbl, "Capacitance in pF"=w403:dbl)  [unwired: 6 in, 2 out]
                                "Capacitance" <- w403
                                "Resistance" <- w402
                                }
                                frame True {
                                n206 = local read "old R Data"() -> (w405:dbl)
                                n207 = local read "old C data"() -> (w404:dbl)
                                }
                                }
                              }
                              frame #5 {
                                n208 = call "SingleStripQuality.vi"("Thresholds"=w409, "Pinhole flag in"=w412, "Resistance Data"=w410, "Capacitance Data"=w411) -> ("Defect Flag"=w408:i32)  [unwired: 2 in, 1 out]
                                n209 = Increment(x=w408) -> (x+1=w407:i32)
                                n210 = To Unsigned Word Integer(number=w407) -> (unsigned 16bit integer=w406:u16)
                                n211 = local write "new flag"(w406) -> ()
                              }
                              frame #6 {
                                n212 = Greater Than 0?(x="Edit Mode:") -> (x > 0?=w413:bool)
                                n213 = local write "Correct Data"(w413) -> ()
                              }
                              frame #7 {
                                n214 = local write "Read"(FALSE ("Read")) -> ()
                              }
                            }
                          }
                        }
                        n215 = local read "go/stop"() -> (w364:bool)
                        n216 = Not(x=w364) -> (.not. x?=w363:bool)
                        n217 = Compound Arithmetic op=OR("Correct Data", "skip this strip", w363) -> (w367:bool)
                        n218 = Not(x=w367) -> (.not. x?=w366:bool)
                      }
                      n219 = case shown="True" w331 {
                        tunnel: w330 -> [_ w333]
                        tunnel: w327 -> [_ w332]
                        frame False {
                        }
                        frame True {
                          n220 = stacked-sequence {
                            tunnel: w333 -> [w336 _]
                            tunnel: w332 -> [w335 w349]
                            frame #0 {
                              w334 = T9."Write Element" ("Action")
                              n221 = local read "new flag"() -> (w339:u16)
                              n222 = Decrement(x=w339) -> (x-1=w338:u16)
                              n223 = local read "Capacitance"() -> (w345:dbl)
                              n224 = local read "Resistance"() -> (w341:dbl)
                              n225 = local read "Current"() -> (w346:dbl)
                              n226 = To Double Precision Float(number=w338) -> (double precision float=w337:dbl)
                              n227 = call "MultiRegionData.vi"("Action"=w334, "Array No."=2, "Array Size / Index"=w336, "Data IN"=w337, "Region index"=w335) -> ()  [unwired: 1 in, 2 out]
                              n228 = call "MultiRegionData.vi"("Action"=w334, "Array No."=1, "Array Size / Index"=w336, "Data IN"=w346, "Region index"=w335) -> ()  [unwired: 1 in, 2 out]
                              n229 = call "MultiRegionData.vi"("Action"=w334, "Array No."=4, "Array Size / Index"=w336, "Data IN"=w341, "Region index"=w335) -> ()  [unwired: 1 in, 2 out]
                              n230 = call "MultiRegionData.vi"("Action"=w334, "Array No."=3, "Array Size / Index"=w336, "Data IN"=w345, "Region index"=w335) -> ()  [unwired: 1 in, 2 out]
                            }
                            frame #1 {
                              n231 = global read "ProbePlanParams.vi" "ProbePlan Parameters IN"() -> (w348:T3)
                              n232 = Unbundle By Name(w348) -> ("Test ProbePoints.Strip length [cm]"=w347:dbl[])
                              n233 = local read "Number of strips probed"() -> (w353:i32)
                              n234 = local read "max scale array"() -> (w357:i32[])
                              n235 = local read "min scale array"() -> (w356:i32[])
                              n236 = local read "Thresholds"() -> (w355:T1)
                              n237 = call "DisplayStriptestData.vi"("Strip Lengths [cm]"=w347, "min scale array"=w356, "max scale array"=w357, "# probed"=w353, "Display Stats?"=TRUE, "Thresholds:"=w355, "Region"=w349) -> ("Resistance [MW]"=w352:cluster{u32, i32, "Array OUT":dbl[]}, "Capacitance [pF]"=w351:cluster{u32, i32, "Array OUT":dbl[]}, "Current [nA]"=w350:cluster{u32, i32, "Array OUT":dbl[]})  [unwired: 2 out]
                              n238 = local write "Current [nA]"(w350) -> ()
                              n239 = local write "Capacitance [pF]"(w351) -> ()
                              n240 = local write "Resistance [MW]"(w352) -> ()
                            }
                          }
                        }
                      }
                    }
                    frame #4 {
                      w416 = FALSE
                      n241 = local write "Read"(w416) -> ()
                      n242 = local write "Correct Data"(w416) -> ()
                    }
                  }
                  n243 = local read "go/stop"() -> (w275:bool)
                  n244 = Not(x=w275) -> (.not. x?=w274:bool)
                  n245 = Greater Or Equal?(x=w283, y=w282) -> (x >= y?=w281:bool)
                  n246 = Not Or(1:w274, 2:w281) -> (0:w280:bool)
                }
              }
              frame #1 {
                w417 = FALSE ("Read")
                n247 = local write "go/stop"(FALSE ("Check strips")) -> ()
                n248 = local write "Read"(w417) -> ()
                n249 = local write "Correct Data"(w417) -> ()
              }
            }
          }
        }
        n250 = case shown="True" "update list" {
          tunnel: w98 -> [w419 w441]
          tunnel: w85 -> [_ w434]
          tunnel: [w419 w435] -> w100
          tunnel: w92 -> [_ w421]
          frame False {
          }
          frame True {
            w424 = T9."Read Array" ("Action")
            n251 = global read "ProbePlanParams.vi" "ProbePlan Parameters IN"() -> (w423:T3)
            n252 = Unbundle By Name(w423) -> ("Test ProbePoints.Strip length [cm]"=w422:dbl[])
            n253 = local read "Thresholds"() -> (w430:T1)
            n254 = call "MultiRegionData.vi"("Action"=w424, "Array No."=3, "Region index"=w421) -> ("Array OUT"=w426:dbl[])  [unwired: 3 in, 1 out]
            n255 = call "MultiRegionData.vi"("Action"=w424, "Array No."=0, "Region index"=w421) -> ("Array OUT"=w425:dbl[])  [unwired: 3 in, 1 out]
            n256 = call "MultiRegionData.vi"("Action"=w424, "Array No."=2, "Region index"=w421) -> ("Array OUT"=w427:dbl[])  [unwired: 3 in, 1 out]
            n257 = call "MultiRegionData.vi"("Action"=w424, "Array No."=4, "Region index"=w421) -> ("Array OUT"=w428:dbl[])  [unwired: 3 in, 1 out]
            n258 = Index Array(array=w422, index=w421) -> (element=w420:dbl)
            n259 = call "StripQuality.vi"("Defect Flag array IN"=w441, "Strip Length [cm]"=w420, "Resistance data array"=w428, "Capacitance Data Array"=w426, "Thresholds:"=w430, "Pinhole flag array in"=w427, "Channel No. Array"=w425, "No of entries"=w434) -> ("Strip Quality Data"=w436:T8)  [unwired: 2 in, 1 out]
            n260 = Unbundle By Name(w436) -> ("No of bad strips"=w429:i32, "Bad channel list"=w432:i32[], "Defect Flag array OUT"=w435:i32[][], "Defect description list"=w433:i32[])
            n261 = call "StripDefectsList.vi"("Defect description list"=w433, "No of strips"=w429, "Bad channel list"=w432) -> ("Defect list"=→"Defects":string)
            n262 = local write "Bad channel list"(w432) -> ()
            n263 = local write "No. of bad channels"(w429) -> ()
          }
        }
      }
    }
    frame #2 {
      w459 = "0"
      n264 = local read "Thresholds"() -> (→"Thresholds copy":T1)
      n265 = global read "QC_MeasurementSetup.vi" "Striptest Measurement Parameters"() -> (w448:T7)
      n266 = Unbundle By Name(w448) -> ("Bias Supply"=w446:refnum<class "SupplyControl.lvclass">, "SMU"=w443:refnum<class "SupplyControl.lvclass">, "ProbeStation"=w447:refnum<class "ProbeStationControl.lvclass">)
      n267 = call-dynamic "Supply_Stby.vi"("SupplyControl in"=w443) -> ("error out"=w442:errorcluster)  [unwired: 9 in, 1 out]
      n268 = local read "Current Bias Voltage [V]"() -> (w452:dbl)
      n269 = call-dynamic "Prober_ChuckUpDown.vi"("error in (no error)"=w442, "Direction"=enum16{"up", "down"}."down", "ProbeStationControl in"=w447) -> ("error out"=w455:errorcluster, "ProbeStationControl out"=w454:refnum<class "ProbeStationControl.lvclass">)  [unwired: 6 in, 1 out]
      n270 = call-dynamic "Prober_MoveToXYZTheta.vi"("Theta location [mdeg]"="none", "ProbeStationControl in"=w454, "error in (no error)"=w455, "Z location [µm]"="down", "Y location [µm]"=w459, "X location [µm]"=w459) -> ("error out"=w453:errorcluster)  [unwired: 3 in, 2 out]
      n271 = call "SupplyRamp.vi"("error in"=w453, "Requested Voltage"=0.0, "Step Size"=10.0, "Step Delay"=1000, "Supply IN"=w446, "Starting Voltage"=w452) -> ("error out"=w445:errorcluster, "Supply OUT"=w444:refnum<class "SupplyControl.lvclass">, "Current Voltage"=w451:dbl)  [unwired: 2 in, 1 out]
      n272 = call-dynamic "Supply_Stby.vi"("error in (no error)"=w445, "SupplyControl in"=w444) -> ()  [unwired: 8 in, 2 out]
      n273 = local write "Current Bias Voltage [V]"(w451) -> ()
    }
  }
  n274 = Unbundle(w3) -> ("Region"=→"Region:":string)  [unwired: 1 out]
